vi "Set Routes.vi"(8 "error in (no error)":errorcluster, 10 "Routes":i32[](array[numeric]), 11 "Mux in":refnum<class "Mux.lvclass">) -> (0 "error out":errorcluster, 3 "Mux out":refnum<class "Mux.lvclass">)   [LabVIEW 2022 SP3, in "VideoMux.lvlib" / "Mux.lvclass"]
uses:
  Mux.lvclass
  Mux.lvclass/Mux.ctl
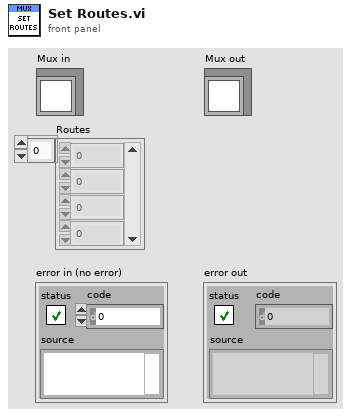
[diagram p1: front panel]
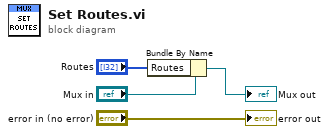
[diagram p0: block diagram]
diagram:
  n1 = Bundle By Name(cluster="Mux in", "Routes"="Routes") -> (→"Mux out":refnum<class "Mux.lvclass">)
  "error out" <- "error in (no error)"
